vi "Update UI Details.vi"(8 "error in":errorcluster, 9 "UI path":path, 10 "measurement service name":string, 11 "project ref":refnum<vi>) -> (0 "error out":errorcluster, 3 "project ref out":refnum<vi>)   [LabVIEW 2021, in "MeasurementService Editor.lvlib"]
uses:
  MeasurementService Editor.lvlib
  <vilib>/Plug-In SDKs/Measurements/Helpers/TypeDefs/User Interface Information.ctl
  <vilib>/Plug-In SDKs/Measurements/NI Measurement Plug-In SDK.lvlib
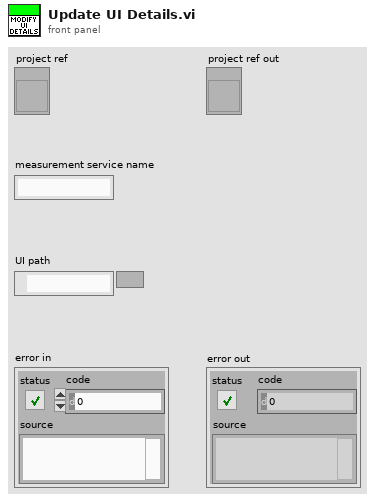
[diagram p1: front panel]
types:
  T1 = typedef "NI Measurement Plug-In SDK.lvlib/User Interface Information.ctl" = cluster{"file":string}
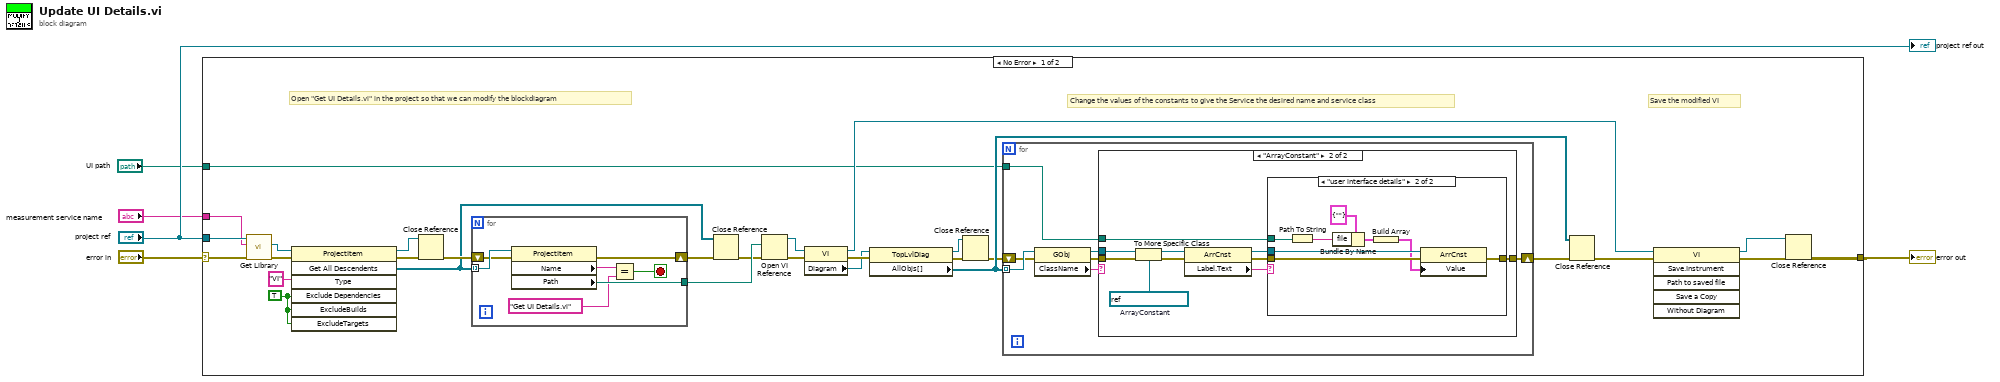
[diagram p0: block diagram]
diagram:
  n1 = case shown="No Error" "error in" {
    selector: "error in" -> [w22 w69]
    tunnel: "project ref" -> [w21 _]
    tunnel: [w32 w69] -> w3
    tunnel: "measurement service name" -> [w15 _]
    tunnel: "UI path" -> [w8 _]
    frame No Error {
      w34 = TRUE ("ExcludeDependencies")
      # "Save the modified VI"
      # "Open \"Get UI Details.vi\" in the project so that we can modify the blockdiagram"
      # "Change the values of the constants to give the Service the desired name and service class"
      n2 = call "Get Library.vi"("error in (no error)"=w22, "library name"=w15, "project ref"=w21) -> ("error out"=w20:errorcluster, "library item"=w19:refnum<vi>)  [unwired: 5 in, 2 out]
      n3 = invoke class="ProjectItem" method="Get All Descendents"(reference=w19, error in=w20, "Type"="VI", "Exclude Dependencies"=w34, "ExcludeBuilds"=w34, "ExcludeTargets"=w34) -> (reference out=w16:refnum<vi>, error out=w18:errorcluster, "All Descendents"=w6:refnum<vi>[])  [unwired: 1 in, 4 out]
      n4 = Close Reference(reference=w16, error in (no error)=w18) -> (error out=w17:errorcluster)
      n5 = for {
        tunnel: w6 -> [w68] mode=indexing
        shift-right: [w63] -> w13
        shift-left: w17 -> [w66]
        tunnel: [w64] -> w14
        stop <- w65 stop-if-true
        n6 = property class="ProjectItem"(reference=w68, error in=w66) -> (error out=w63:errorcluster, "Name"=w67:string, "Path"=w64:path)  [unwired: 1 out]
        n7 = Equal?(x=w67, y="Get UI Details.vi") -> (x = y?=w65:bool)
      }
      n8 = Close Reference(reference=w6, error in (no error)=w13) -> (error out=w7:errorcluster)
      n9 = Open VI Reference(vi path=w14, error in (no error)=w7) -> (vi reference=w29:refnum<vi>, error out=w27:errorcluster)  [unwired: 4 in]
      n10 = property class="VI"(reference=w29, error in=w27) -> (reference out=w25:refnum<vi>, error out=w28:errorcluster, "Diagram"=w26:refnum<vi>)
      n11 = property class="TopLvlDiag"(reference=w26, error in=w28) -> (reference out=w9:refnum<vi>, error out=w11:errorcluster, "AllObjs[]"=w12:refnum<vi>[])
      n12 = Close Reference(reference=w9, error in (no error)=w11) -> (error out=w10:errorcluster)
      n13 = for {
        tunnel: w12 -> [w41] mode=indexing
        shift-right: [w37] -> w24
        shift-left: w10 -> [w40]
        tunnel: w8 -> [w35]
        n14 = property class="GObj"(reference=w41, error in=w40) -> (reference out=w39:refnum<vi>, error out=w38:errorcluster, "ClassName"=w36:string)
        n15 = case shown="\"ArrayConstant\"" w36 {
          tunnel: w39 -> [_ w51]
          tunnel: w38 -> [w42 w50]
          tunnel: w35 -> [_ w49]
          tunnel: [w42 w48] -> w37
          frame Default {
          }
          frame "ArrayConstant" {
            w52 = refnum<vi> refnum  # ArrayConstant
            n16 = To More Specific Class(target class=w52, reference=w51, error in=w50) -> (specific class reference=w47:refnum<vi>, error out=w46:errorcluster)
            n17 = property class="ArrCnst"(reference=w47, error in=w46) -> (reference out=w45:refnum<vi>, error out=w44:errorcluster, "Label.Text"=w43:string)
            n18 = case shown="\"user interface details\"" w43 {
              tunnel: w49 -> [_ w55]
              tunnel: [w53 w61] -> w48
              tunnel: w45 -> [_ w60]
              tunnel: w44 -> [w53 w59]
              frame Default {
              }
              frame "user interface details" {
                n19 = Path To String(path=w55) -> (string=w54:string)
                n20 = Bundle By Name(cluster=T1 {"file"=""} ("UI Information"), "file"=w54) -> (w57:T1)
                n21 = Build Array(w57) -> (w56:T1[])
                n22 = property class="ArrCnst"(reference=w60, error in=w59, "Value"=w56) -> (error out=w61:errorcluster)  [unwired: 1 out]
              }
            }
          }
        }
      }
      n23 = Close Reference(reference=w12, error in (no error)=w24) -> (error out=w23:errorcluster)
      n24 = invoke class="VI" method="Save.Instrument"(reference=w25, error in=w23) -> (reference out=w31:refnum<vi>, error out=w30:errorcluster)  [unwired: 4 in, 4 out]
      n25 = Close Reference(reference=w31, error in (no error)=w30) -> (error out=w32:errorcluster)
    }
    frame Error {
    }
  }
  "error out" <- w3
  "project ref out" <- "project ref"
